vi "LivePosition.vi"() -> ()   [LabVIEW 2015]
uses:
  <vilib>/Platform/TimedLoop/XDataNode/timing_clust.ctl
  <vilib>/Platform/TimedLoop/XDataNode/nitl_modes.ctl
  <vilib>/Platform/TimedLoop/XDataNode/wakeup.ctl
  <vilib>/Platform/TimedLoop/XDataNode/XDataNode.xnode
  <vilib>/Platform/TimedLoop/XDataNode/XDNodeRunTimeDep.lvlib
  <userlib>/Newport ESP301/Newport ESP301.lvlib
panel:
  in  "stop 2":bool
  out "Axis 3 Pos.":dbl
  out "Axis 2 Pos.":dbl
  out "Axis 1 Pos.":dbl
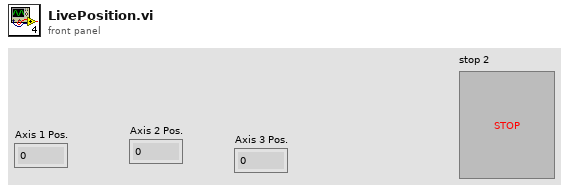
[diagram p1: front panel]
types:
  T1 = typedef "XDNodeRunTimeDep.lvlib/timing_clust.ctl" = cluster{"Expected End [f-1]":u64, "Actual End [f-1]":u64, "Finished Late? [f-1]":bool, "Expected End [i-1]":u64, "Actual End [i-1]":u64, "Finished Late? [i-1]":bool, "Expected Start [i]":u64, "Actual Start [i]":u64, "Expected Start [f]":u64, "Actual Start [f]":u64, "Source Name":string, "Structure Name":string, "Period":i64, "Deadline":i64, "Offset":i64, "Start":i64, "Priority":i32, "Timeout":i32, "Mode":T2, "Wakeup Reason":T3, "Error":errorcluster, "Source Type":string, "Secondary Source Type":string, "Global End Time":u64, "Global Start Time":u64, "Frame Duration":u64, "Iteration Duration":u64, "Assigned CPU":i32, "I/O Scan Engine Mode":u32}
  T2 = typedef "XDNodeRunTimeDep.lvlib/nitl_modes.ctl" = enum32{"No Change", "Process missed periods, maintain original phase", "Discard missed periods, maintain original phase", "Process missed periods, ignore original phase", "Discard missed periods, ignore original phase"}
  T3 = typedef "XDNodeRunTimeDep.lvlib/wakeup.ctl" = enum32{"Normal", "Aborted", "Asynchronous wakeup", "Timing source error", "Timed loop error", "Timeout"}
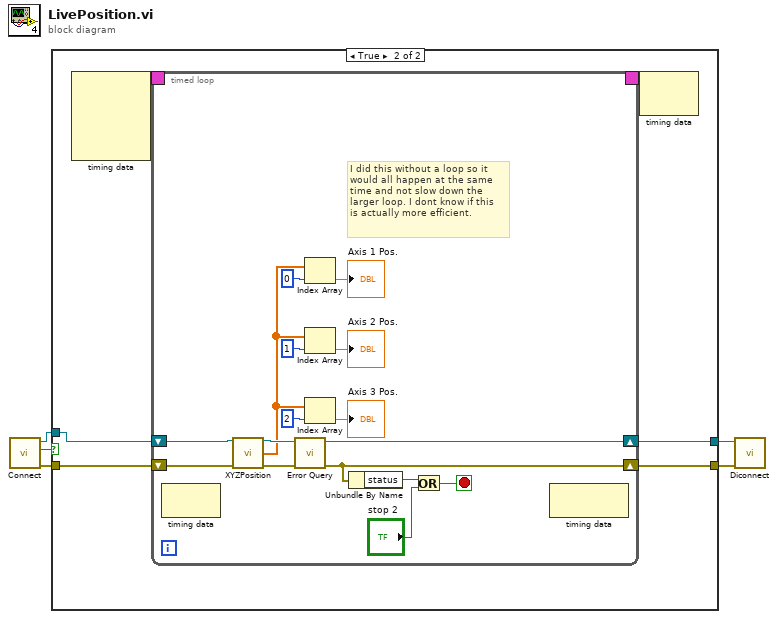
[diagram p0: block diagram]
diagram:
  n1 = call "Connect.vi"() -> ("error out"=w3:errorcluster, "Connected"=w4:bool, "VISA resource name out"=w5:refnum<visa-resource-name>)  [unwired: 5 in]
  n2 = case shown="True" w4 {
    tunnel: [w7 w13] -> w2
    tunnel: [w6 w12] -> w1
    tunnel: w5 -> [w7 w11]
    tunnel: w3 -> [w6 w10]
    frame False {
    }
    frame True {
      n3 = node-c288() -> (w9:T1)  [unwired: 4 in]
      n4 = timed-loop {
        timing: w9 -> [_]
        timing-out: [_] -> w8
        shift-right: [w25] -> w13
        shift-left: w11 -> [w29]
        shift-right: [w23] -> w12
        shift-left: w10 -> [w28]
        stop <- w21 stop-if-true
        # "I did this without a loop so it\nwould all happen at the same \ntime and not slow down the \nlarger loop. I dont know if this\nis actually more efficient."
        n5 = node-c288() -> ()  [unwired: 1 in, 1 out]
        n6 = call "XYZPosition.vi"("VISA resource name"=w29, "error in"=w28) -> ("VISA resource name out"=w26:refnum<visa-resource-name>, "[x,y,z]"=w20:dbl[], "error out"=w27:errorcluster)  [unwired: 11 in]
        n7 = call <userlib>:"Error Query.vi"("error in (no error)"=w27, "VISA resource name"=w26) -> ("error out"=w23:errorcluster, "VISA resource name out"=w25:refnum<visa-resource-name>)  [unwired: 2 in, 2 out]
        n8 = Index Array(array=w20, index=0) -> (element=→"Axis 1 Pos.":dbl)
        n9 = Index Array(array=w20, index=1) -> (element=→"Axis 2 Pos.":dbl)
        n10 = Index Array(array=w20, index=2) -> (element=→"Axis 3 Pos.":dbl)
        n11 = Unbundle By Name(w23) -> ("status"=w22:bool)
        n12 = Or(x=w22, y="stop 2") -> (x .or. y?=w21:bool)
        n13 = node-c288() -> ()  [unwired: 1 in, 1 out]
      }
      n14 = node-c288(w8) -> ()  [unwired: 1 out]
    }
  }
  n15 = call "Diconnect.vi"("error in (no error)"=w1, "VISA resource name"=w2) -> ()  [unwired: 6 in]
